vi "To and From String Array Test.vi"() -> (0 "error out":errorcluster, 2 "Pass":bool)   [LabVIEW 2015, in "Tests.lvlib"]
uses:
  Tests.lvlib
  Config/Wait Step Config.lvclass
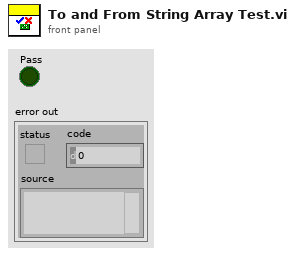
[diagram p1: front panel]
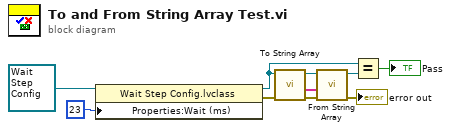
[diagram p0: block diagram]
diagram:
  n1 = property class="Wait Step Config.lvclass"(reference=refnum<class "Wait Step Config.lvclass"> refnum ("Wait Step Config.lvclass"), "Properties:Wait (ms)"=u32 23 ("Wait (ms)")) -> (reference out=w3:refnum<class "Wait Step Config.lvclass">, error out=w8:errorcluster)  [unwired: 1 in]
  n2 = call-dynamic "To String Array.vi"("error in (no error)"=w8, "Wait Step Config in"=w3) -> ("error out"=w7:errorcluster, "Step String Array"=w5:string[], "Wait Step Config out"=w6:refnum<class "Wait Step Config.lvclass">)  [unwired: 7 in]
  n3 = call-dynamic "From String Array.vi"("error in (no error)"=w7, "String Array"=w5, "Wait Step Config in"=w6) -> ("error out"=→"error out":errorcluster, "Wait Step Config out"=w4:refnum<class "Wait Step Config.lvclass">)  [unwired: 7 in]
  n4 = Equal?(x=w3, y=w4) -> (x = y?=→"Pass":bool)
